vi "Decode LoFlo Status Errors.vi"(0 "Status":u8[](array[numeric]) format="%x") -> (1 "CO2 Errors":string[](array[string]), 2 "Zero Status":T1(ring), 3 "Zero In Process":bool, 4 "Zero Required":bool)   [LabVIEW 2016]
panel:
  out "ComboBox Errors":string[](array[combo])
  out "Numeric":i32
  out "Numeric 2":i32
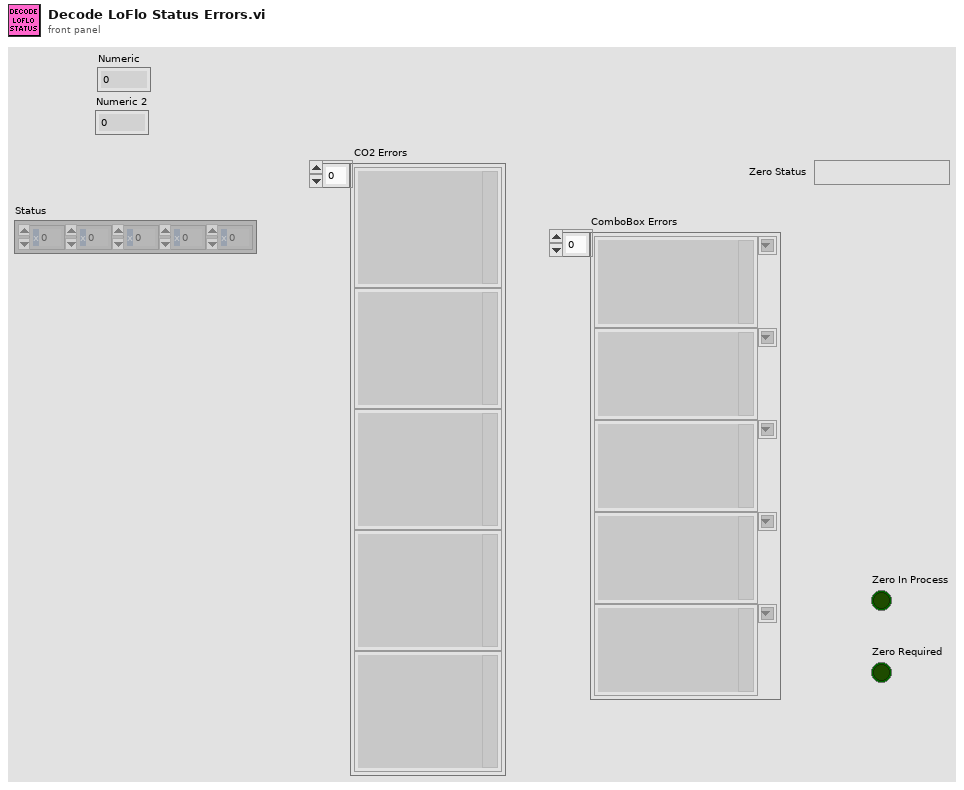
[diagram p1: front panel]
types:
  T1 = enum16{" ", "Zero In Progress", "Zero Required", "Zero Error"}
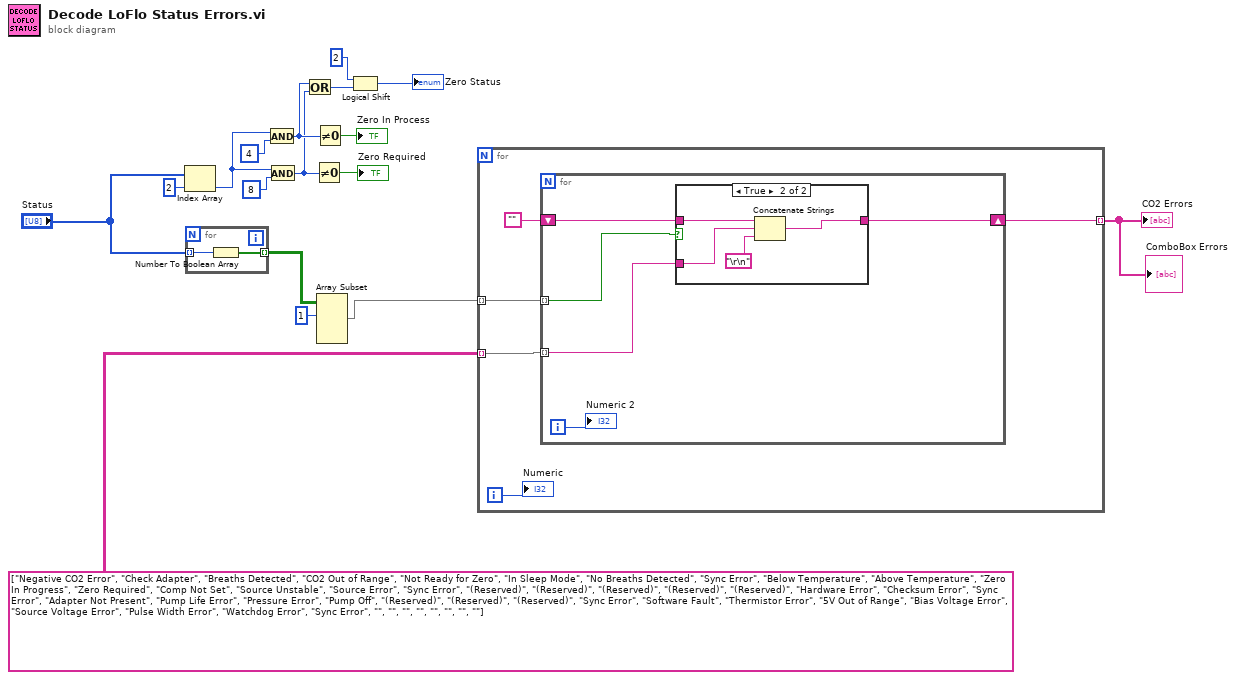
[diagram p0: block diagram]
diagram:
  n1 = Index Array(array="Status", index=2) -> (element=w8:u8)
  n2 = for {
    tunnel: "Status" -> [w19] mode=indexing
    tunnel: [w18] -> w13 mode=indexing
    n3 = Number To Boolean Array(number=w19) -> (Boolean array=w18:bool[])
  }
  n4 = And(x=w8, y=u8 4) -> (x .and. y?=w3:u8)
  n5 = And(x=w8, y=u8 8) -> (x .and. y?=w2:u8)
  n6 = Or(x=w3, y=w2) -> (x .or. y?=w4:u8)
  n7 = Not Equal To 0?(x=w2) -> (x != 0?=→"Zero Required":bool)
  n8 = Not Equal To 0?(x=w3) -> (x != 0?=→"Zero In Process":bool)
  n9 = Array Subset(array=w13, index (row)=1 ("index")) -> (w14:bool[][])  [unwired: 3 in]
  n10 = Logical Shift(y=i16 2, x=w4) -> (x << y=→"Zero Status":u8)
  n11 = for {
    tunnel: w14 -> [w23] mode=indexing
    tunnel: string[][] [["Negative CO2 Error", "Check Adapter", "Breaths Detected", "CO2 Out of Range", "Not Ready for Zero", "In Sleep Mode", "No Breaths Detected", "Sync Error"], ["Below Temperature", "Above Temperature", "Zero In Progress", "Zero Required", "Comp Not Set", "Source Unstable", "Source Error", "Sync Error"], ["(Reserved)", "(Reserved)", "(Reserved)", "(Reserved)", "(Reserved)", "Hardware Error", "Checksum Error", "Sync Error"], ["Adapter Not Present", "Pump Life Error", "Pressure Error", "Pump Off", "(Reserved)", "(Reserved)", "(Reserved)", "Sync Error"], ["Software Fault", "Thermistor Error", "5V Out of Range", "Bias Voltage Error", "Source Voltage Error", "Pulse Width Error", "Watchdog Error", "Sync Error"], ["", "", "", "", "", "", "", ""]] -> [w22] mode=indexing
    tunnel: [w20] -> w16 mode=indexing
    i -> [w24]
    n12 = for {
      tunnel: w23 -> [w28] mode=indexing
      tunnel: w22 -> [w26] mode=indexing
      shift-right: [w25] -> w20
      shift-left: "" -> [w27]
      i -> [w29]
      n13 = case shown="True" w28 {
        tunnel: w27 -> [w30 w34]
        tunnel: w26 -> [_ w33]
        tunnel: [w30 w31] -> w25
        frame False {
        }
        frame True {
          n14 = Concatenate Strings(w34, w33, "\r\n") -> (w31:string)
        }
      }
      "Numeric 2" <- w29
    }
    "Numeric" <- w24
  }
  "CO2 Errors" <- w16
  "ComboBox Errors" <- w16
